vi "QPlus_Lockin_External Reference - Copy.vi"() -> ()   [LabVIEW 2016]
uses:
  <instrlib>/Stanford Research 830/Public/Data/Read (1 Parameter).vi
  <vilib>/Utility/file.llb/Write Delimited Spreadsheet (DBL).vi
  <instrlib>/Stanford Research 830/Stanford Research 830.lvlib
  <instrlib>/Agilent 3352X Series/Agilent 3352X Series.lvlib
panel:
  in  "Reference name":refnum<visa-resource-name>
  out "FWHM":dbl
  out "Quality Factor":dbl
  out "Integrated Signal":cluster{"Y":dbl[], "Y":dbl[]}[](graph)
  out "Resonance Frequency":dbl
  in  "VISA resource name":refnum<visa-resource-name>
  in  "Sensitivity (26: 1 V/uA)":i8(ring)=26 items=["Auto Gain"=-1, "2 nV/fA"=0, "5 nV/fA"=1, "10 nV/fA"=2, "20 nV/fA"=3, "50 nV/fA"=4, "100 nV/fA"=5, "200 nV/fA"=6, "500 nV/fA"=7, "1 uV/pA"=8, "2 uV/pA"=9, "5 uV/pA"=10, "10 uV/pA"=11, "20 uV/pA"=12, "50 uV/pA"=13, "100 uV/pA"=14, "200 uV/pA"=15, "500 uV/pA"=16, "1 mV/nA"=17, "2 mV/nA"=18, "5 mV/nA"=19, "10 mV/nA"=20, "20 mV/nA"=21, "50 mV/nA"=22, "100 mV/nA"=23, "200 mV/nA"=24, "500 mV/mA"=25, "1 V/uA"=26]
  in  "Time Constant (8: 100ms)":u16(ring)=8 items=["10 us", "30 us", "100 us", "300 us", "1 ms", "3 ms", "10 ms", "30 ms", "100 ms", "300 ms", "1 s", "3 s", "10 s", "30 s", "100 s", "300 s", "1 ks", "3 ks", "10 ks", "30 ks"]
  out "Raw Signal":cluster{"Y":dbl[], "Y":dbl[]}[](graph)
  in  "Save File Name":path=path "G:/UCB/Instruments/tip making/Qplus AFM tip making/qplus test/Caihong/CJ39.xlsx" caption="Filename"
  in  "Time Between Points (sec)":dbl=0.05 format="%#_1f"
  in  "Sine Output Amplitude (1 V)":dbl=1.0
  in  "Starting Frequency (Hz)":dbl=32000.0
  in  "Final Frequency (Hz)":dbl=33000.0
  in  "Step Size (Hz)":dbl=10.0
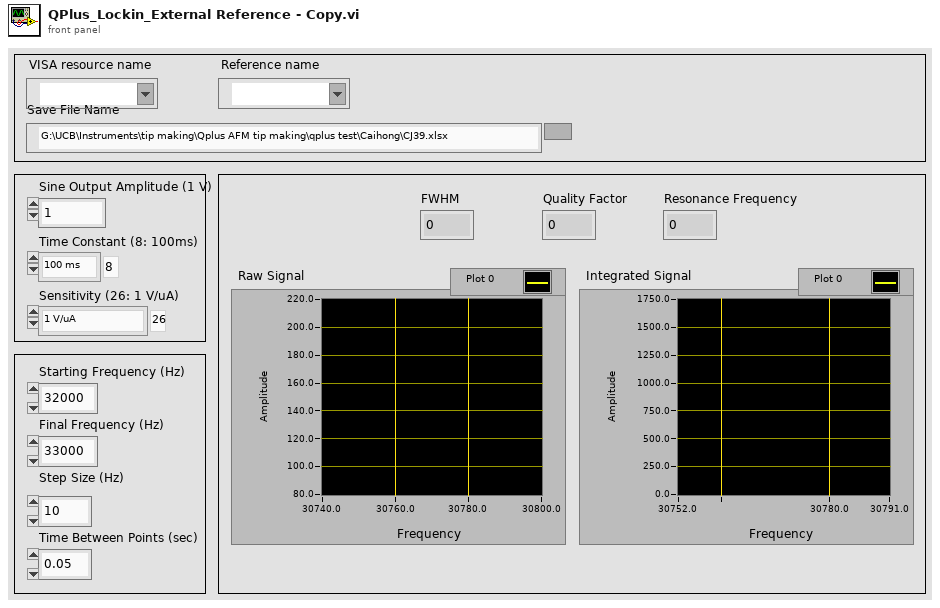
[diagram p1: front panel]
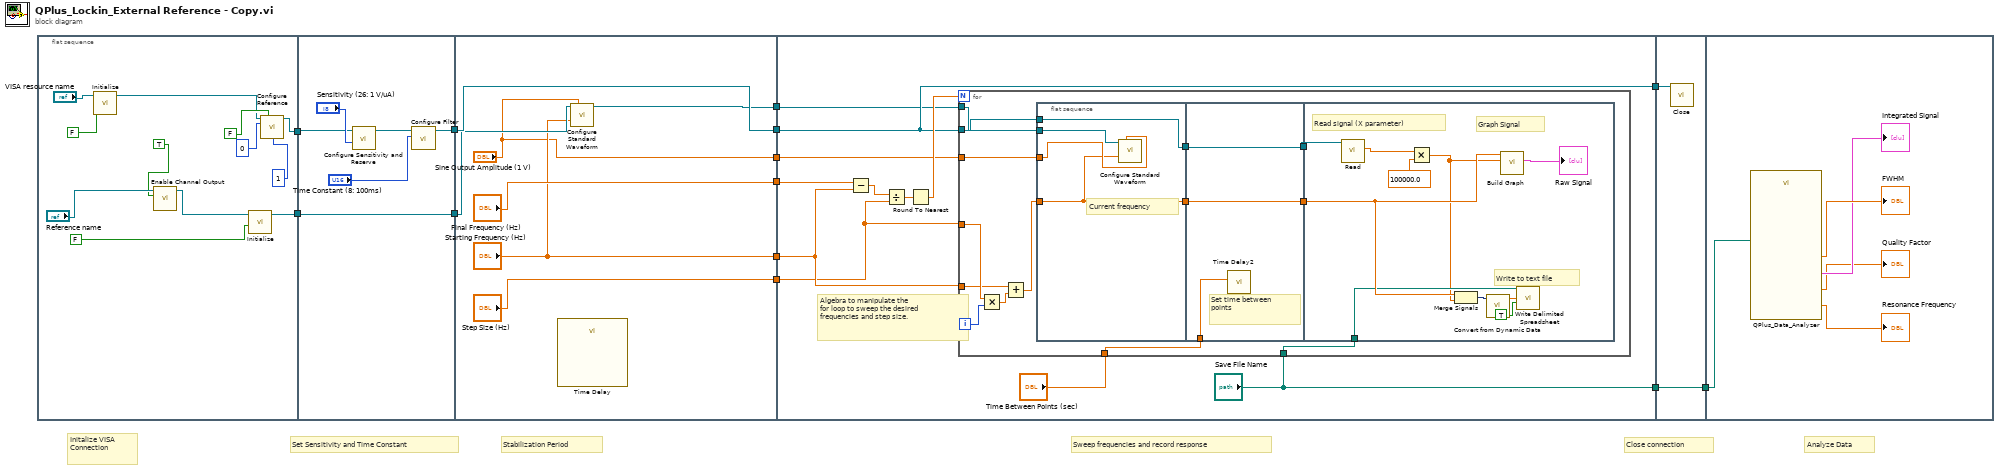
[diagram p0: block diagram]
diagram:
  # "Stabilization Period"
  # "Analyze Data"
  # "Close connection"
  # "Sweep frequencies and record response"
  # "Set Sensitivity and Time Constant"
  # "Initalize VISA\nConnection"
  n1 = flat-sequence {
    tunnel: [w21] -> w13
    tunnel: [w22] -> w2
    tunnel: [w28] -> w9
    tunnel: w13 -> [w27]
    tunnel: [w26] -> w3
    tunnel: w2 -> [w26]
    tunnel: w9 -> [w36]
    tunnel: [w36] -> w8
    tunnel: ["Starting Frequency (Hz)"] -> w7
    tunnel: ["Final Frequency (Hz)"] -> w6
    tunnel: ["Step Size (Hz)"] -> w5
    tunnel: ["Sine Output Amplitude (1 V)"] -> w4
    tunnel: w3 -> [w34]
    tunnel: [w35] -> w1
    tunnel: w8 -> [w46]
    tunnel: [w46] -> w12
    tunnel: ["Save File Name"] -> w11
    tunnel: w7 -> [w43]
    tunnel: w6 -> [w42]
    tunnel: w5 -> [w41]
    tunnel: w4 -> [w40]
    tunnel: w1 -> [w39]
    tunnel: w12 -> [w82]
    tunnel: w11 -> [w81]
    tunnel: [w81] -> w10
    tunnel: w10 -> [w87]
    frame #0 {
      n2 = call <instrlib>:"Initialize.vi"("Reset (True)"=FALSE, "VISA resource name"="VISA resource name") -> ("VISA resource name out"=w14:refnum<visa-resource-name>)  [unwired: 8 in, 1 out]
      n3 = call <instrlib>:"Enable Channel Output.vi"("Enable Output (T: Enable)"=TRUE, "VISA resource name"="Reference name") -> ("VISA resource name out"=w16:refnum<visa-resource-name>)  [unwired: 8 in, 1 out]
      n4 = call <instrlib>:"Initialize.vi"("Reset (Enable)"=FALSE, "VISA resource name"=w16) -> ("VISA resource name out"=w22:refnum<visa-resource-name>)  [unwired: 8 in, 1 out]
      n5 = call "Configure Reference.vi"("VISA resource name"=w14, "Auto Phase (T: Enabled)"=FALSE, "Reference Source (1: Internal)"=0, "External Reference Trigger (0: Sine Zero Crossing)"=1) -> ("VISA resource name out"=w21:refnum<visa-resource-name>)  [unwired: 10 in, 1 out]
    }
    frame #1 {
      n6 = call <instrlib>:"Configure Sensitivity and Reserve.vi"("Sensitivity (-1: Auto gain)"="Sensitivity (26: 1 V/uA)", "VISA resource name"=w27) -> ("VISA resource name out"=w30:refnum<visa-resource-name>)  [unwired: 8 in, 1 out]
      n7 = call <instrlib>:"Configure Filter.vi"("Time Constant (8: 100ms)"="Time Constant (8: 100ms)", "VISA resource name"=w30) -> ("VISA resource name out"=w28:refnum<visa-resource-name>)  [unwired: 8 in, 1 out]
    }
    frame #2 {
      n8 = call "Time Delay"() -> ()  [unwired: 11 in, 1 out]
      n9 = call <instrlib>:"Configure Standard Waveform.vi"("VISA resource name"=w34, "Amplitude (0.1 Vpp)"="Sine Output Amplitude (1 V)", "Frequency/Sample Rate/Bandwidth (1000 Hz)"="Starting Frequency (Hz)") -> ("VISA resource name out"=w35:refnum<visa-resource-name>)  [unwired: 11 in, 1 out]
    }
    frame #3 {
      # "Algebra to manipulate the\nfor loop to sweep the desired\nfrequencies and step size."
      n10 = Subtract(x=w42, y=w43) -> (x-y=w49:dbl)
      n11 = Divide(x=w49, y=w41) -> (x/y=w48:dbl)
      n12 = Round To Nearest(number=w48) -> (nearest integer value=w47:dbl)
      n13 = for {
        N: w47 -> [_]
        tunnel: w41 -> [w62]
        tunnel: w43 -> [w60]
        tunnel: w46 -> [w51]
        tunnel: "Time Between Points (sec)" -> [w53]
        tunnel: "Save File Name" -> [w58]
        tunnel: w40 -> [w57]
        tunnel: w39 -> [w52]
        i -> [w63]
        n14 = Multiply(x=w62, y=w63) -> (x*y=w61:dbl)
        n15 = Add(x=w60, y=w61) -> (x+y=w59:dbl)
        n16 = flat-sequence {
          tunnel: [w64] -> w55
          tunnel: w59 -> [w64]
          tunnel: w57 -> [w66]
          tunnel: w52 -> [w65]
          tunnel: w51 -> [w67]
          tunnel: [w67] -> w50
          tunnel: [w70] -> w56
          tunnel: w55 -> [w69]
          tunnel: [w69] -> w54
          tunnel: w53 -> [w68]
          tunnel: w50 -> [w70]
          tunnel: w56 -> [w76]
          tunnel: w54 -> [w75]
          tunnel: w58 -> [w74]
          frame #0 {
            # "Current frequency"
            n17 = call <instrlib>:"Configure Standard Waveform.vi"("VISA resource name"=w65, "Amplitude (0.1 Vpp)"=w66, "Frequency/Sample Rate/Bandwidth (1000 Hz)"=w64) -> ()  [unwired: 11 in, 2 out]
          }
          frame #1 {
            # "Set time between\npoints"
            n18 = call "Time Delay2"("Delay Time (s)"=w68) -> ()  [unwired: 10 in, 1 out]
          }
          frame #2 {
            # "Read signal (X parameter)"
            # "Graph Signal"
            # "Write to text file"
            n19 = call-poly <instrlib>:"Read.vi"("VISA resource name"=w76) -> ("Measurement"=w73:dbl)  [unwired: 8 in, 2 out]
            n20 = Multiply(x=w73, y=100000.0) -> (x*y=w71:dbl)
            n21 = Merge Signals(w75, w71) -> (w78:dynamicdata)
            n22 = call "Convert from Dynamic Data"("Dynamic Data Type"=w78) -> ("Array"=w77:dbl[])  [unwired: 3 in]
            n23 = call "Build Graph"("Y Input"=w71, "X Input"=w75) -> ("XY Graph"=→"Raw Signal":cluster{"Y":dbl[], "Y":dbl[]}[])  [unwired: 3 in, 6 out]
            n24 = call-poly <vilib>:"Write Delimited Spreadsheet.vi"("file path (dialog if empty)"=w74, "1D data"=w77, "append to file? (new file:F)"=TRUE) -> ()  [unwired: 11 in, 2 out]
          }
        }
      }
    }
    frame #4 {
      n25 = call <instrlib>:"Close.vi"("VISA resource name"=w82) -> ()  [unwired: 10 in, 1 out]
    }
    frame #5 {
      n26 = call "QPlus_Data_Analyzer.vi"("File Path"=w87) -> ("Resonance Frequency"=→"Resonance Frequency":dbl, "Quality Factor"=→"Quality Factor":dbl, "FWHM"=→"FWHM":dbl, "Integrated Signal"=→"Integrated Signal":cluster{"Y":dbl[], "Y":dbl[]}[])  [unwired: 7 in]
    }
  }
